vi "TCP_test.vi"() -> ()   [LabVIEW 2020]
panel:
  out "TCP error":errorcluster
  out "Data length":i32
  in  "ToPC":string="123456789"
  out "FromPC":string
  in  "Strat":bool
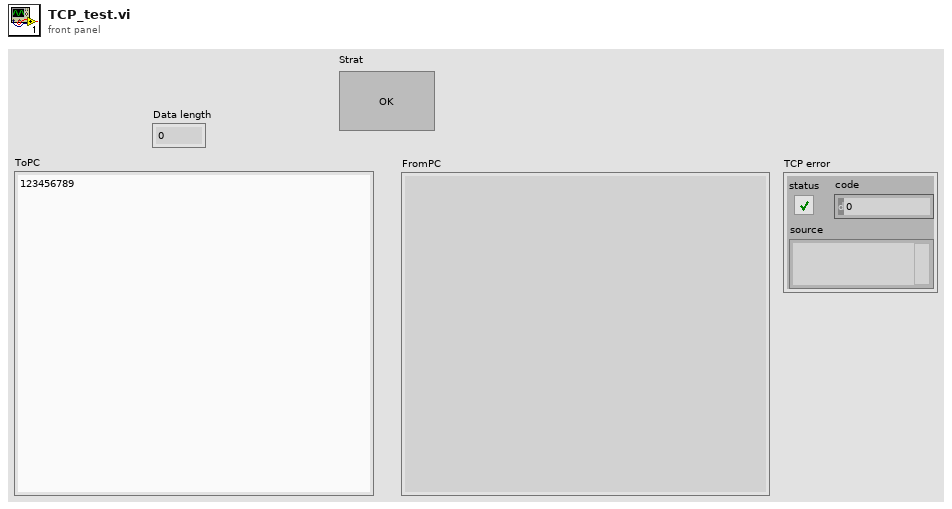
[diagram p1: front panel]
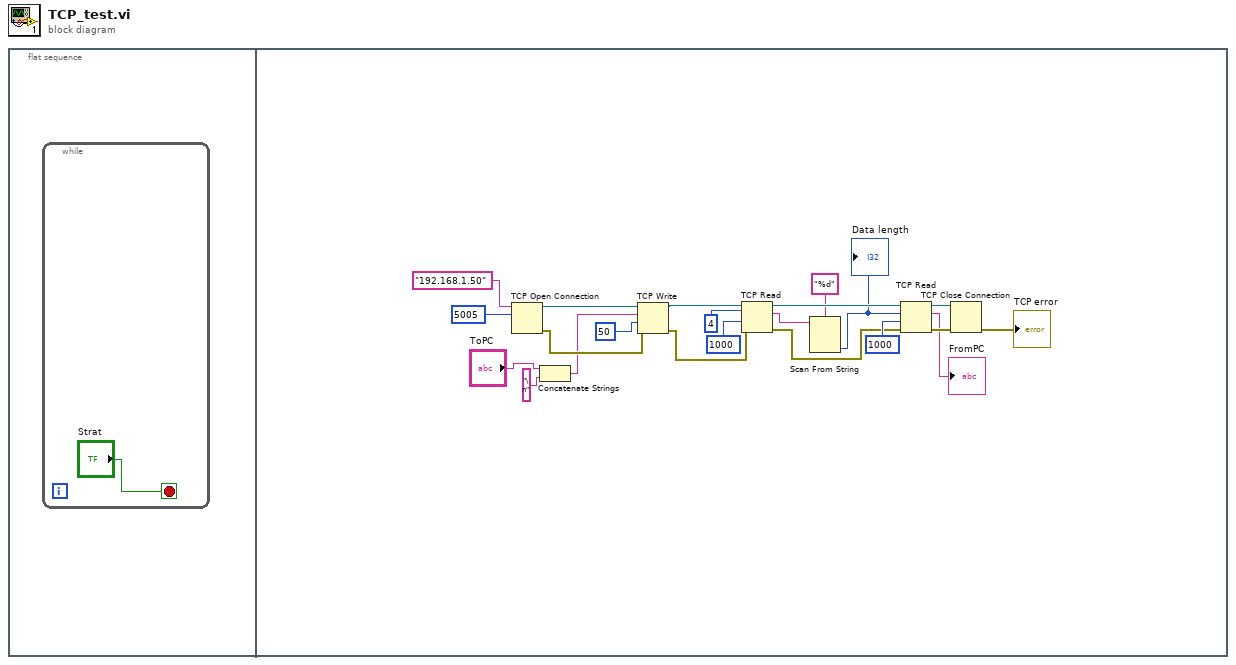
[diagram p0: block diagram]
diagram:
  n1 = flat-sequence {
    frame #0 {
      n2 = while {
        stop <- "Strat" stop-if-true
      }
    }
    frame #1 {
      n3 = TCP Open Connection(address="192.168.1.50", remote port or service name=u16 5005) -> (connection ID=w21:refnum<k5>, error out=w11:errorcluster)  [unwired: 3 in]
      n4 = Concatenate Strings("ToPC", "\n" ("string")) -> (w2:string)
      n5 = TCP Write(connection ID=w21, data in=w2, error in (no error)=w11, 9:50 ("timeout ms (25000)")) -> (connection ID out=w12:refnum<k5>, error out=w10:errorcluster)  [unwired: 1 out]
      n6 = TCP Read(connection ID=w12, bytes to read=4, error in (no error)=w10, 9:1000 ("timeout ms (25000)")) -> (connection ID out=w16:refnum<k5>, data out=w15:string, error out=w13:errorcluster)  [unwired: 1 in]
      n7 = Scan From String(format string="%d", input string=w15) -> (output 1=w6:i32)  [unwired: 3 in, 3 out]
      "Data length" <- w6
      n8 = TCP Read(connection ID=w16, bytes to read=w6, error in (no error)=w13, 9:1000 ("timeout ms (25000)")) -> (connection ID out=w9:refnum<k5>, data out=→"FromPC":string, error out=w8:errorcluster)  [unwired: 1 in]
      n9 = TCP Close Connection(connection ID=w9, error in (no error)=w8) -> (error out=→"TCP error":errorcluster)  [unwired: 1 in, 1 out]
    }
  }
